vi "SFCS_Input_OperatorID.vi"() -> ()   [LabVIEW 2011]
uses:
  Instance           9 29Saved   SFCS_Input_OperatorID .vi
  data/MCSDLL.dll
  Instance           6 29Saved   SFCS_Input_OperatorID .vi
  Instance           8 29Saved   SFCS_Input_OperatorID .vi
  <vilib>/regexp/Match Regular Expression.xnode
panel:
  out "OP ID":string caption="請輸入工號 Input OP ID"
  out "軟體版本 Software Version":string
  out "begin time":u32
  out "Project_NAME":string
  out "URL":string
  # "你的工號:請TE 在MCS Server 先定義\nPC 的網線需接好"
  # "請輸入你的工號\nPlease Input Your ID"
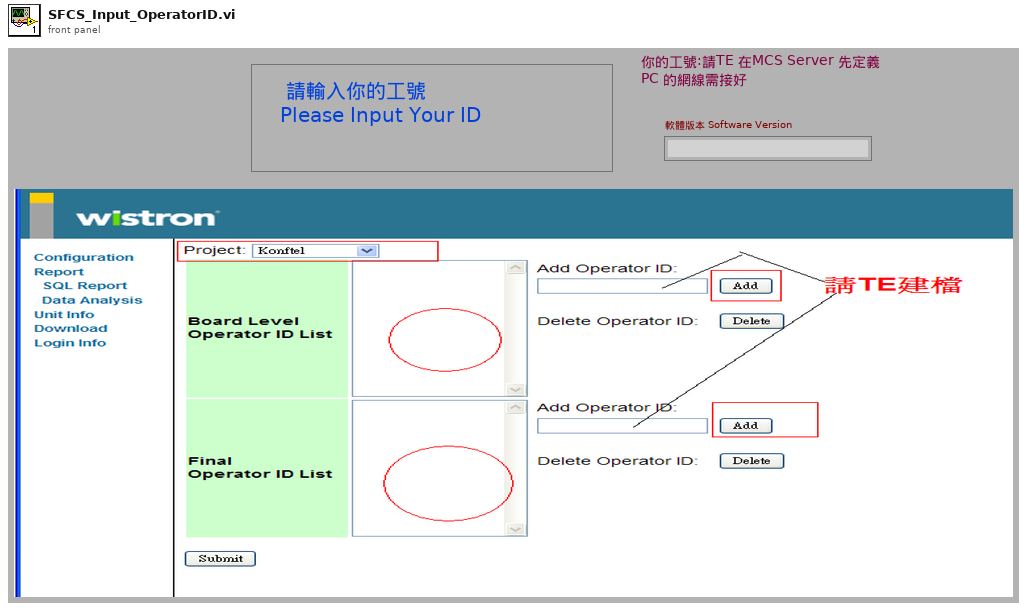
[diagram p1: front panel]
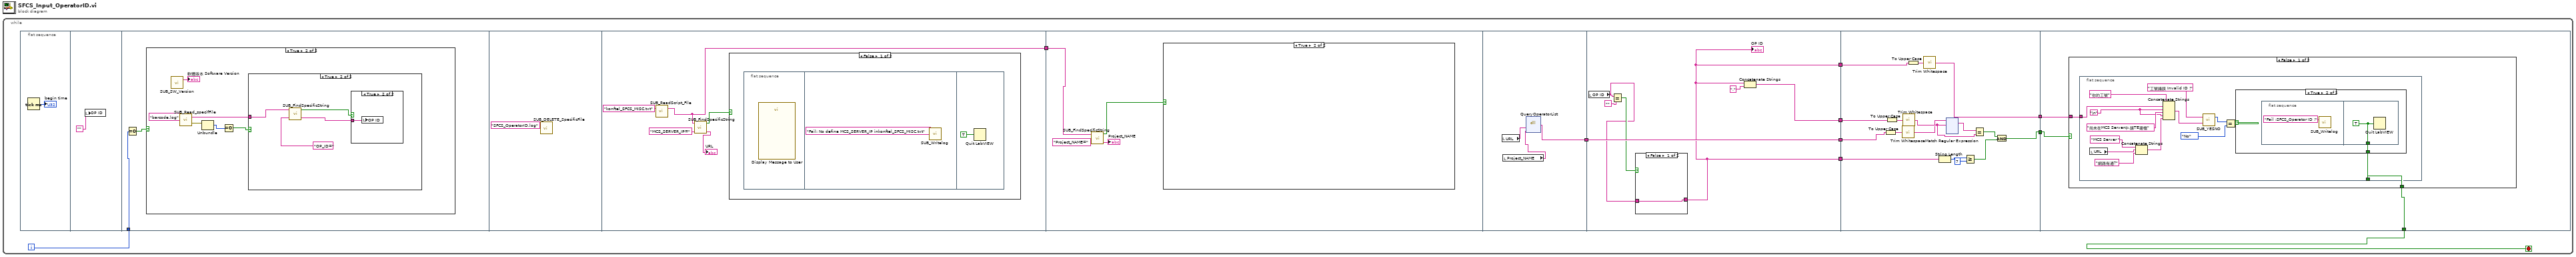
[diagram p0: block diagram]
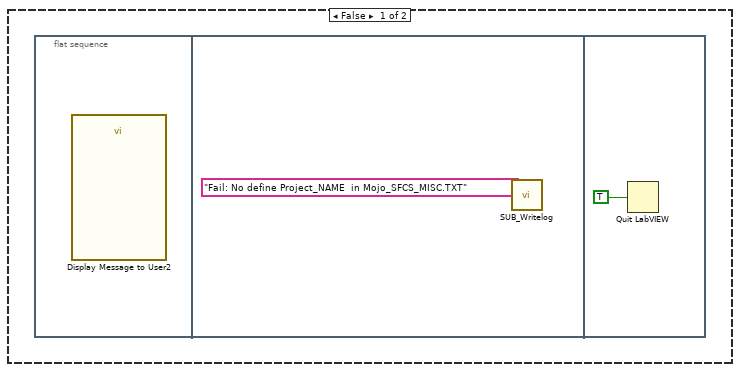
[diagram p6: hidden frame]
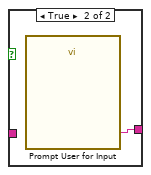
[diagram p7: hidden frame]
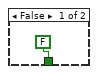
[diagram p8: hidden frame]
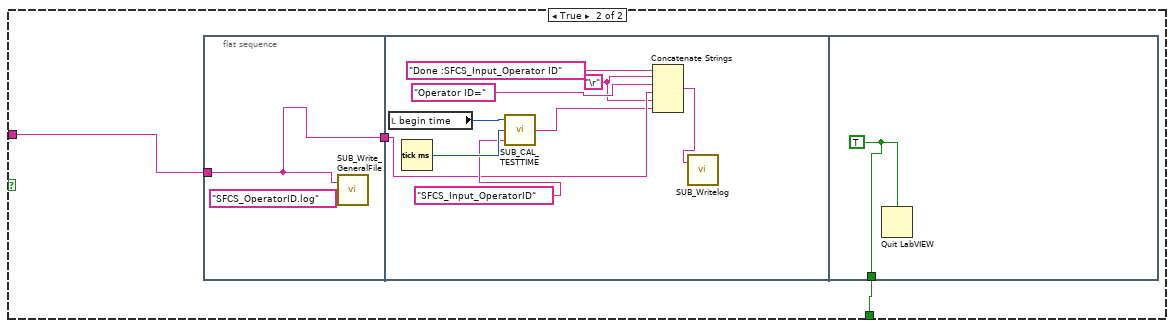
[diagram p9: hidden frame]
diagram:
  n1 = while {
    i -> [w2]
    stop <- w10 stop-if-true
    n2 = flat-sequence {
      tunnel: w2 -> [w14]
      tunnel: [w28] -> w9
      tunnel: w9 -> [w35]
      tunnel: [w40] -> w1
      tunnel: [w49] -> w8
      tunnel: w1 -> [w49]
      tunnel: [w47] -> w6
      tunnel: [w44] -> w5
      tunnel: [w44] -> w4
      tunnel: w8 -> [w65]
      tunnel: [w60] -> w7
      tunnel: w6 -> [w59]
      tunnel: w5 -> [w58]
      tunnel: w4 -> [w53]
      tunnel: [w52] -> w3
      tunnel: [w181] -> w10
      tunnel: w7 -> [w180]
      tunnel: w3 -> [w179]
      frame #0 {
        n3 = Tick Count (ms)() -> (millisecond timer value=→"begin time":u32)
      }
      frame #1 {
        n4 = local write "OP ID"("") -> ()
      }
      frame #2 {
        n5 = Equal To 0?(x=w14) -> (x = 0?=w13:bool)
        n6 = case shown="True" w13 {
          frame False {
          }
          frame True {
            n7 = call "SUB_SW_Version.vi"() -> ("Current Software Version"=→"軟體版本 Software Version":string)  [unwired: 3 in]
            n8 = call "SUB_Read_specifFile.vi"("name or relative path"="barcode.log") -> ("error out"=w19:errorcluster, "text"=w16:string)  [unwired: 1 in]
            n9 = Unbundle(w19) -> ("code"=w20:i32)  [unwired: 2 out]
            n10 = Equal To 0?(x=w20) -> (x = 0?=w17:bool)
            n11 = case shown="True" w17 {
              tunnel: w16 -> [_ w23]
              frame False {
              }
              frame True {
                n12 = call "SUB_FindSpecificString.vi"("Find this String"="OP_ID=", "String data"=w23) -> ("before \"; \" string"=w21:string, "Found"=w22:bool)  [unwired: 2 in]
                n13 = case shown="True" w22 {
                  tunnel: w21 -> [_ w25]
                  frame False {
                  }
                  frame True {
                    n14 = local write "OP ID"(w25) -> ()
                  }
                }
              }
            }
          }
        }
      }
      frame #3 {
        n15 = call "SUB_DELETE_SpecificFile.vi"("Filename to be  Deleted"="SFCS_OperatorID.log") -> ()  [unwired: 2 in, 1 out]
      }
      frame #4 {
        n16 = call "SUB_ReadScript_File.vi"("Script FileName"="konftel_SFCS_MISC.txt") -> ("text"=w28:string)  [unwired: 1 in, 1 out]
        n17 = call "SUB_FindSpecificString.vi"("Find this String"="MCS_SERVER_IP=", "String data"=w28) -> ("before \"; \" string"=→"URL":string, "Found"=w29:bool)  [unwired: 2 in]
        n18 = case shown="False" w29 {
          frame False {
            n19 = flat-sequence {
              frame #0 {
                n20 = call "Display Message to User"() -> ()  [unwired: 10 in, 2 out]
              }
              frame #1 {
                n21 = call "SUB_Writelog.vi"("Pass/Fail"="Fail: No define MCS_SERVER_IP inkonftel_SFCS_MISC.txt") -> ()  [unwired: 2 in]
              }
              frame #2 {
                n22 = Quit LabVIEW(quit? (T)=TRUE) -> ()
              }
            }
          }
          frame True {
          }
        }
      }
      frame #5 {
        n23 = call "SUB_FindSpecificString.vi"("Find this String"="Project_NAME=", "String data"=w35) -> ("before \"; \" string"=→"Project_NAME":string, "Found"=w36:bool)  [unwired: 2 in]
        n24 = case shown="True" w36 {
          frame False {
            n25 = flat-sequence {
              frame #0 {
                n26 = call "Display Message to User2"() -> ()  [unwired: 10 in, 2 out]
              }
              frame #1 {
                n27 = call "SUB_Writelog.vi"("Pass/Fail"="Fail: No define Project_NAME  in Mojo_SFCS_MISC.TXT") -> ()  [unwired: 2 in]
              }
              frame #2 {
                n28 = Quit LabVIEW(quit? (T)=TRUE) -> ()
              }
            }
          }
          frame True {
          }
        }
      }
      frame #6 {
        n29 = local read "URL"() -> (w42:string)
        n30 = local read "Project_NAME"() -> (w41:string)
        n31 = dll-call lib="D:/S8300E_Project/data/MCSDLL.dll" fn="QueryOperatorList" label="Call Library Function Node"("URL"=w42, "ProjectName"=w41) -> (w40:string)  [unwired: 5 in, 2 out]
      }
      frame #7 {
        n32 = local read "OP ID"() -> (w43:string)
        n33 = Equal?(x=w43, y="") -> (x = y?=w45:bool)
        n34 = case shown="False" w45 {
          tunnel: [w50 w51] -> w44
          tunnel: w43 -> [w50 _]
          frame False {
          }
          frame True {
            n35 = call "Prompt User for Input"() -> ("請輸入工號 Input OP ID"=w51:string)  [unwired: 17 in, 2 out]
          }
        }
        "OP ID" <- w44
        n36 = Concatenate Strings(w44, ",") -> (w47:string)
      }
      frame #8 {
        n37 = To Upper Case(1:w65) -> (0:w66:string)
        n38 = To Upper Case(1:w59) -> (0:w67:string)
        n39 = call <vilib>:"Trim Whitespace.vi"("string"=w66) -> ("trimmed string"=w62:string)  [unwired: 1 in]
        n40 = call <vilib>:"Trim Whitespace.vi"("string"=w67) -> ("trimmed string"=w63:string)  [unwired: 1 in]
        n41 = To Upper Case(1:w53) -> (0:w54:string)
        n42 = call <vilib>:"Trim Whitespace.vi"("string"=w54) -> ("trimmed string"=w52:string)  [unwired: 1 in]
        n43 = String Length(string=w58) -> (length=w57:i32)
        n44 = xnode "Match Regular Expression"("input string"=w62, "regular expression"=w63) -> ("whole match"=w64:string)  [unwired: 4 in, 4 out]
        n45 = Greater Or Equal?(x=w57, y=7) -> (x >= y?=w55:bool)
        n46 = Equal?(x=w64, y=w63) -> (x = y?=w61:bool)
        n47 = And(x=w61, y=w55) -> (x .and. y?=w60:bool)
      }
      frame #9 {
        n48 = case shown="False" w180 {
          tunnel: [w183 w204] -> w181
          tunnel: w179 -> [w182 w203]
          frame False {
            n49 = flat-sequence {
              tunnel: [w193] -> w183
              tunnel: w182 -> [w191]
              frame #0 {
                w188 = "\n"
                n50 = local read "URL"() -> (w186:string)
                n51 = Concatenate Strings("MCS Server " ("string"), w186, "網路有通?" ("string")) -> (w184:string)
                n52 = Concatenate Strings("你的工號", w191, w188, "尚未在MCS Server中,請TE建檔", w188, w184) -> (w190:string)
                n53 = call "SUB_YESNO.vi"("Debug View"=w190, "Status"="工號錯誤 Invalid ID !") -> ("yes/no"=w196:enum32{"No Selection", "Yes", "No", "None"})  [unwired: 1 in]
                n54 = Equal?(x=w196, y=enum32{"No Selection", "Yes", "No", "None"}."No") -> (x = y?=w194:bool)
                n55 = case shown="True" w194 {
                  tunnel: [FALSE ("quit? (T)") w199] -> w193
                  frame False {
                  }
                  frame True {
                    n56 = flat-sequence {
                      tunnel: [w201] -> w199
                      frame #0 {
                        n57 = call "SUB_Writelog.vi"("Pass/Fail"="Fail :SFCS_Operator ID !") -> ()  [unwired: 2 in]
                      }
                      frame #1 {
                        w201 = TRUE ("quit? (T)")
                        n58 = Quit LabVIEW(quit? (T)=w201) -> ()
                      }
                    }
                  }
                }
              }
            }
          }
          frame True {
            n59 = flat-sequence {
              tunnel: w203 -> [w205]
              tunnel: [w205] -> w202
              tunnel: w202 -> [w210]
              tunnel: [w216] -> w204
              frame #0 {
                n60 = call "SUB_Write_GeneralFile.vi"("Filename"="SFCS_OperatorID.log", "Text Input"=w205) -> ()  [unwired: 1 out]
              }
              frame #1 {
                w209 = "\r"
                n61 = local read "begin time"() -> (w215:u32)
                n62 = Tick Count (ms)() -> (millisecond timer value=w214:u32)
                n63 = call "SUB_CAL_TESTTIME.vi"("Test Item name"="SFCS_Input_OperatorID", "Stop tick time"=w214, "Start tick time"=w215) -> ("Test Time output"=w208:string)  [unwired: 2 in]
                n64 = Concatenate Strings("Done :SFCS_Input_Operator ID" ("Pass/Fail"), w209, "Operator ID=" ("string"), w210, w209, w208) -> (w207:string)
                n65 = call "SUB_Writelog.vi"("Pass/Fail"=w207) -> ()  [unwired: 2 in]
              }
              frame #2 {
                w216 = TRUE ("quit? (T)")
                n66 = Quit LabVIEW(quit? (T)=w216) -> ()
              }
            }
          }
        }
      }
    }
  }
